vi "GobangServer_contents.vi"   [LabVIEW 2014, in "GoBang.lvlib"]
uses:
  GoBang.lvlib
  CS++GoBangServer.lvclass
  CS++GoBangServer Messages/Update Connection State Msg/Update Connection State Msg.lvclass
  CS++GoBangServer Messages/Analyse Board Msg/Analyse Board Msg.lvclass
  CS++GoBangServer Messages/JoinGame Msg/JoinGame Msg.lvclass
  CS++GoBangServer Messages/Reset Board Msg/Reset Board Msg.lvclass
  LNA_GoBang/LNA_GoBang.lvclass
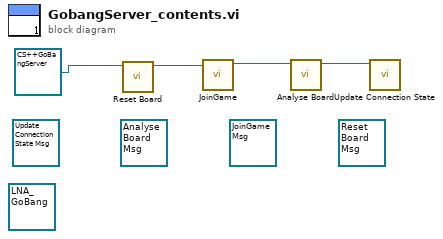
[diagram p0: block diagram]
diagram:
  (unwired) refnum<class "LNA_GoBang.lvclass"> refnum ("GoBang.lvlib:LNA_GoBang.lvclass")
  (unwired) refnum<class "Reset Board Msg.lvclass"> refnum ("GoBang.lvlib:Reset Board Msg.lvclass")
  (unwired) refnum<class "JoinGame Msg.lvclass"> refnum ("GoBang.lvlib:JoinGame Msg.lvclass")
  (unwired) refnum<class "Analyse Board Msg.lvclass"> refnum ("GoBang.lvlib:Analyse Board Msg.lvclass")
  (unwired) refnum<class "Update Connection State Msg.lvclass"> refnum ("GoBang.lvlib:Update Connection State Msg.lvclass")
  n1 = call-dynamic "Reset Board.vi"("CS++GoBangServer in"=refnum<class "CS++GoBangServer.lvclass"> refnum ("GoBang.lvlib:CS++GoBangServer.lvclass")) -> ("CS++GoBangServer out"=w3:refnum<class "CS++GoBangServer.lvclass">)  [unwired: 9 in, 1 out]
  n2 = call-dynamic "JoinGame.vi"("CS++GoBangServer in"=w3) -> ("CS++GoBangServer out"=w2:refnum<class "CS++GoBangServer.lvclass">)  [unwired: 9 in, 1 out]
  n3 = call-dynamic "Analyse Board.vi"("CS++GoBangServer in"=w2) -> ("CS++GoBangServer out"=w1:refnum<class "CS++GoBangServer.lvclass">)  [unwired: 9 in, 1 out]
  n4 = call-dynamic "Update Connection State.vi"("CS++GoBangServer in"=w1) -> ()  [unwired: 9 in, 2 out]
